vi "music_pictures_by_index.set.vi"(8 "error in (no error)":errorcluster, 10 "Music Pictures by Index":T1(c390), 11 "midi-ui in":refnum<class "midi-ui.lvclass">) -> (0 "error out":errorcluster, 3 "midi-ui out":refnum<class "midi-ui.lvclass">)   [LabVIEW 2020, in "midi-ui.lvclass"]
uses:
  midi-ui.lvclass
  midi-ui.lvclass/midi-ui.ctl
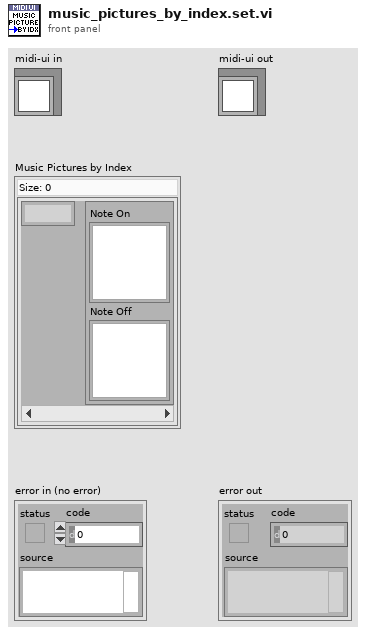
[diagram p1: front panel]
types:
  T1 = map{i32, cluster{"Note On":picture, "Note Off":picture}}
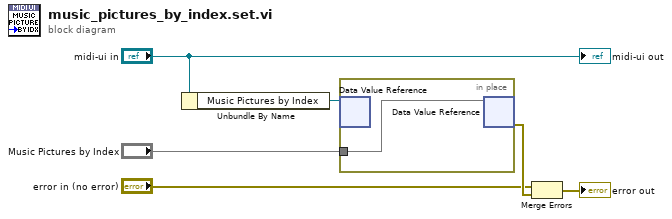
[diagram p0: block diagram]
diagram:
  n1 = Unbundle By Name("midi-ui in") -> ("Music Pictures by Index"=w6:refnum<data-value>)
  n2 = in-place {
    in-place-border: "Music Pictures by Index" -> [w7]
    n3 = in-place-dvr #1(w6) -> ()  [unwired: 2 out]
    n4 = in-place-dvr #1(w7) -> (w4:errorcluster)  [unwired: 1 out]
  }
  n5 = Merge Errors("error in (no error)", w4) -> (→"error out":errorcluster)
  "midi-ui out" <- "midi-ui in"
